vi "data_analysis main.vi"() -> ()   [LabVIEW 2017]
uses:
  <vilib>/Analysis/baseanly.llb/Mean (DBL).vi
  <vilib>/Waveform/WDTFileIO.llb/Export Waveforms To Spreadsheet File (1D).vi
  <vilib>/Analysis/NI_AALBase.lvlib
panel:
  out "x/y":dbl
  out "Zmag trajectory":waveform(dbl) caption="元素"
  out "Ext.":dbl
  out "Z pos":waveform(dbl)(graph)
  out "Zmag pos":waveform(dbl)(graph)
  out "data name":string
  out "cursor pos":dbl
  out "cursor length":dbl
  out "zmag cursor pos":dbl
  out "zmag cursor length":dbl
  out "current bead":string
  in  "graphs":enum32{"raw data", "force calculation"}(tab)
  out "XY图":cluster{dbl[], dbl[]}(graph)
  in  "ref NO.":i32 min=0
  in  "remove drift":bool
  in  "sample rate":dbl=200.0
  in  "zero point offset":bool
  out "x_0":dbl caption="X0" format="%0.2f"
  out "y_0":dbl caption="Y0" format="%0.2f"
  out "z_0":dbl caption="Z0" format="%0.2f"
  in  "file save path":path
  in  "数据另存为":bool
  in  "data type":enum16{"tdms", "gr", "excel"}(ring)
  out "保存完成？":bool
  in  "停止":bool
  in  "file path":path
  in  "load data":bool
  in  "data info":i32(listbox)
  in  "bead NO.":i32 min=0
  in  "trajectory":i32 min=0
  out "Z mag":dbl
  in  "zmag or force":enum32{"zmag", "force"}(radio)
  out "array of strings":string[](array[string])
  out "string":string
  in  "doubleFace?":bool
  in  "B":dbl=-1.436
  in  "A":dbl=142.6
  in  "cali source":enum32{"X", "Y"}(radio)
  out "Power spectrum (um^2/Hz)":cluster{dbl[], "Spectrum out":dbl[]}[](graph)
  in  "Z_shift":dbl
  out "Force graph":cluster{dbl[], dbl[]}(graph)
  in  "accept":bool
  in  "force estimate":bool
  in  "Fit settings":T1={"#PSD Averages"=40, "Correct camera acquisition artifacts"=TRUE, "Autorange"=TRUE, "fstart (Hz)"=0.0, "Pendulum geometry"=FALSE, "Fit model"=FALSE} {"#PSD Averages" min=1}
  in  "fsampling (Hz)":dbl=2800.0
  in  "DNA length (um)":dbl=0.658
  out "Fit Results":T2
  out "fit data":dbl[][](array[numeric])
  # "load force-zmag"
  # "F="
  # "exp(                *Zmag)"
  # "*"
  # "Fit parameters"
  # "Calculated quantities"
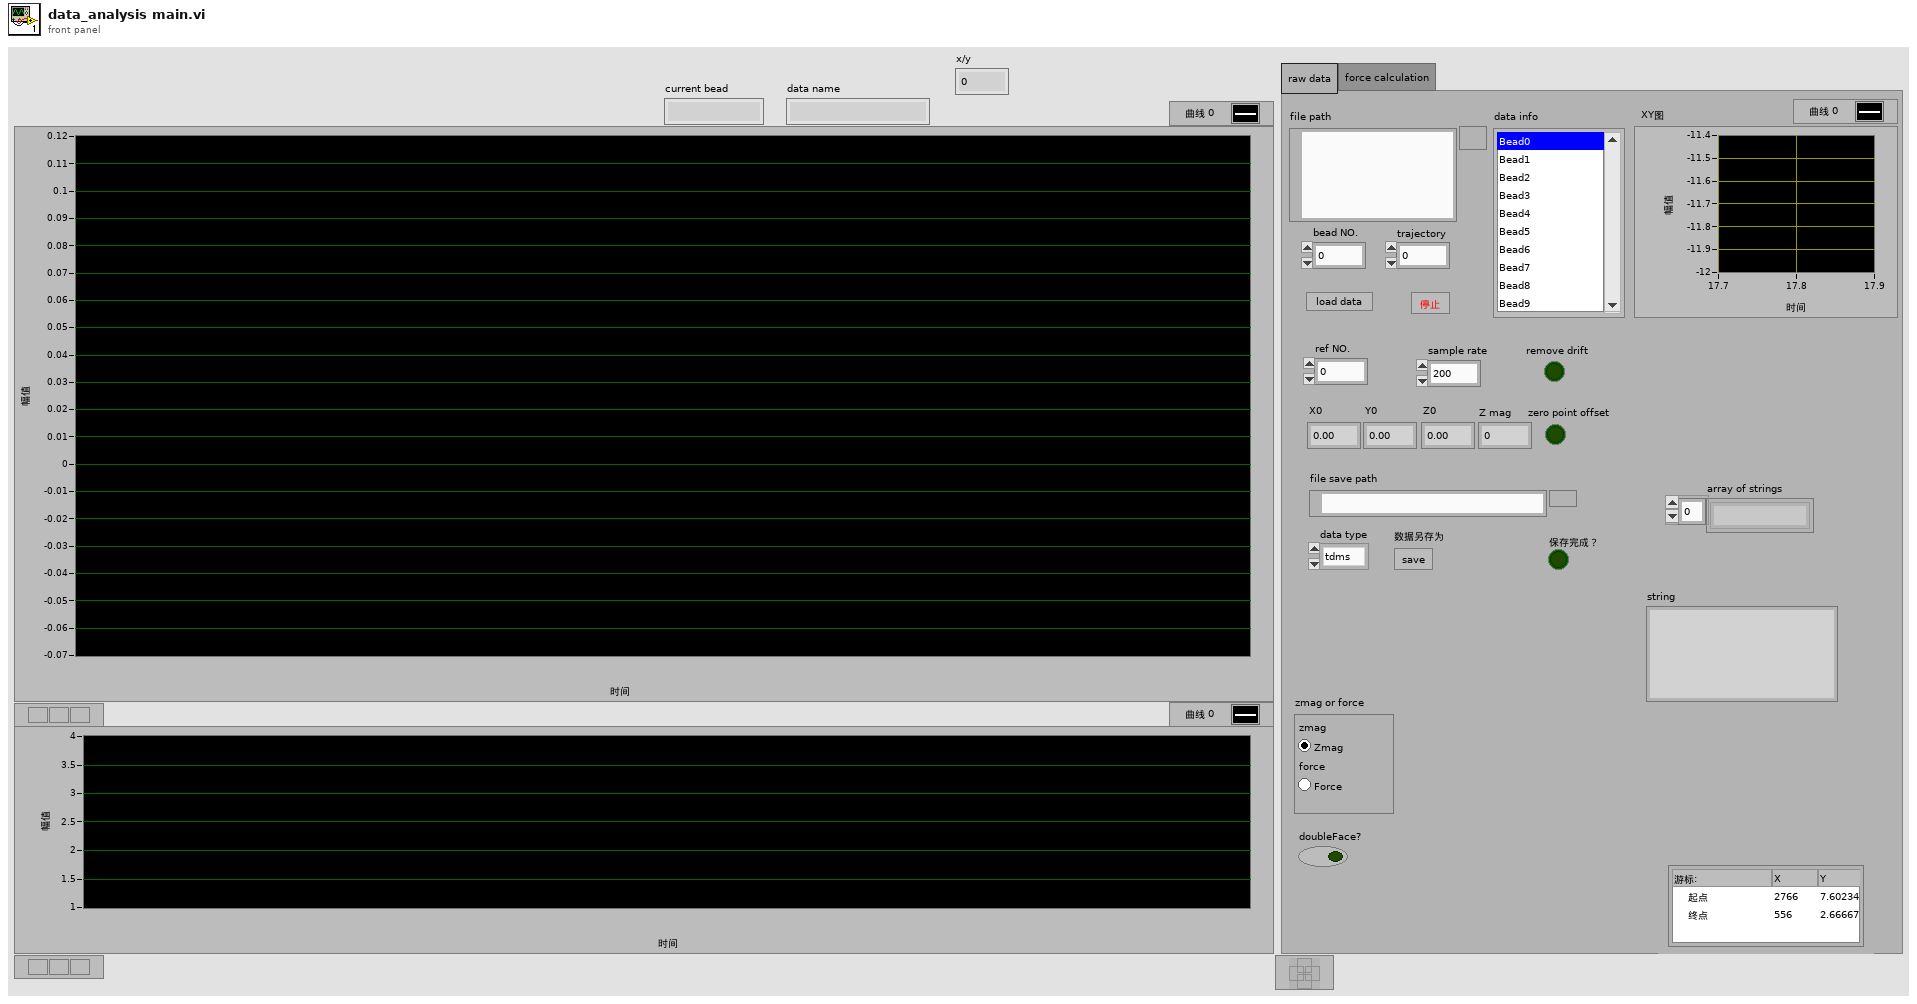
[diagram p1: front panel]
types:
  T1 = cluster{"#PSD Averages":u8, "Correct camera acquisition artifacts":bool, "Autorange":bool, "fstart (Hz)":dbl, "Pendulum geometry":bool, "Fit model":bool}
  T2 = cluster{"fcut (Hz)":dbl, "x2 (µm^2)":dbl, "Force (pN)":dbl, "Radius (µm)":dbl, "Apparent hydrodyn. radius (µm)":dbl, "fcut Error (Hz)":dbl, "x2 Error (µm^2)":dbl, "Force Error (pN)":dbl, "Radius Error (µm)":dbl, "Residue (unbiased)":dbl, "In range?":bool}
  T3 = enum16{"open", "open or create", "create or replace", "create", "open (read-only)"}
  T4 = enum16{"big-endian, network order", "native, host order", "little-endian"}
  T5 = enum16{"open", "replace", "create", "open or create", "replace or create", "replace or create with confirmation"}
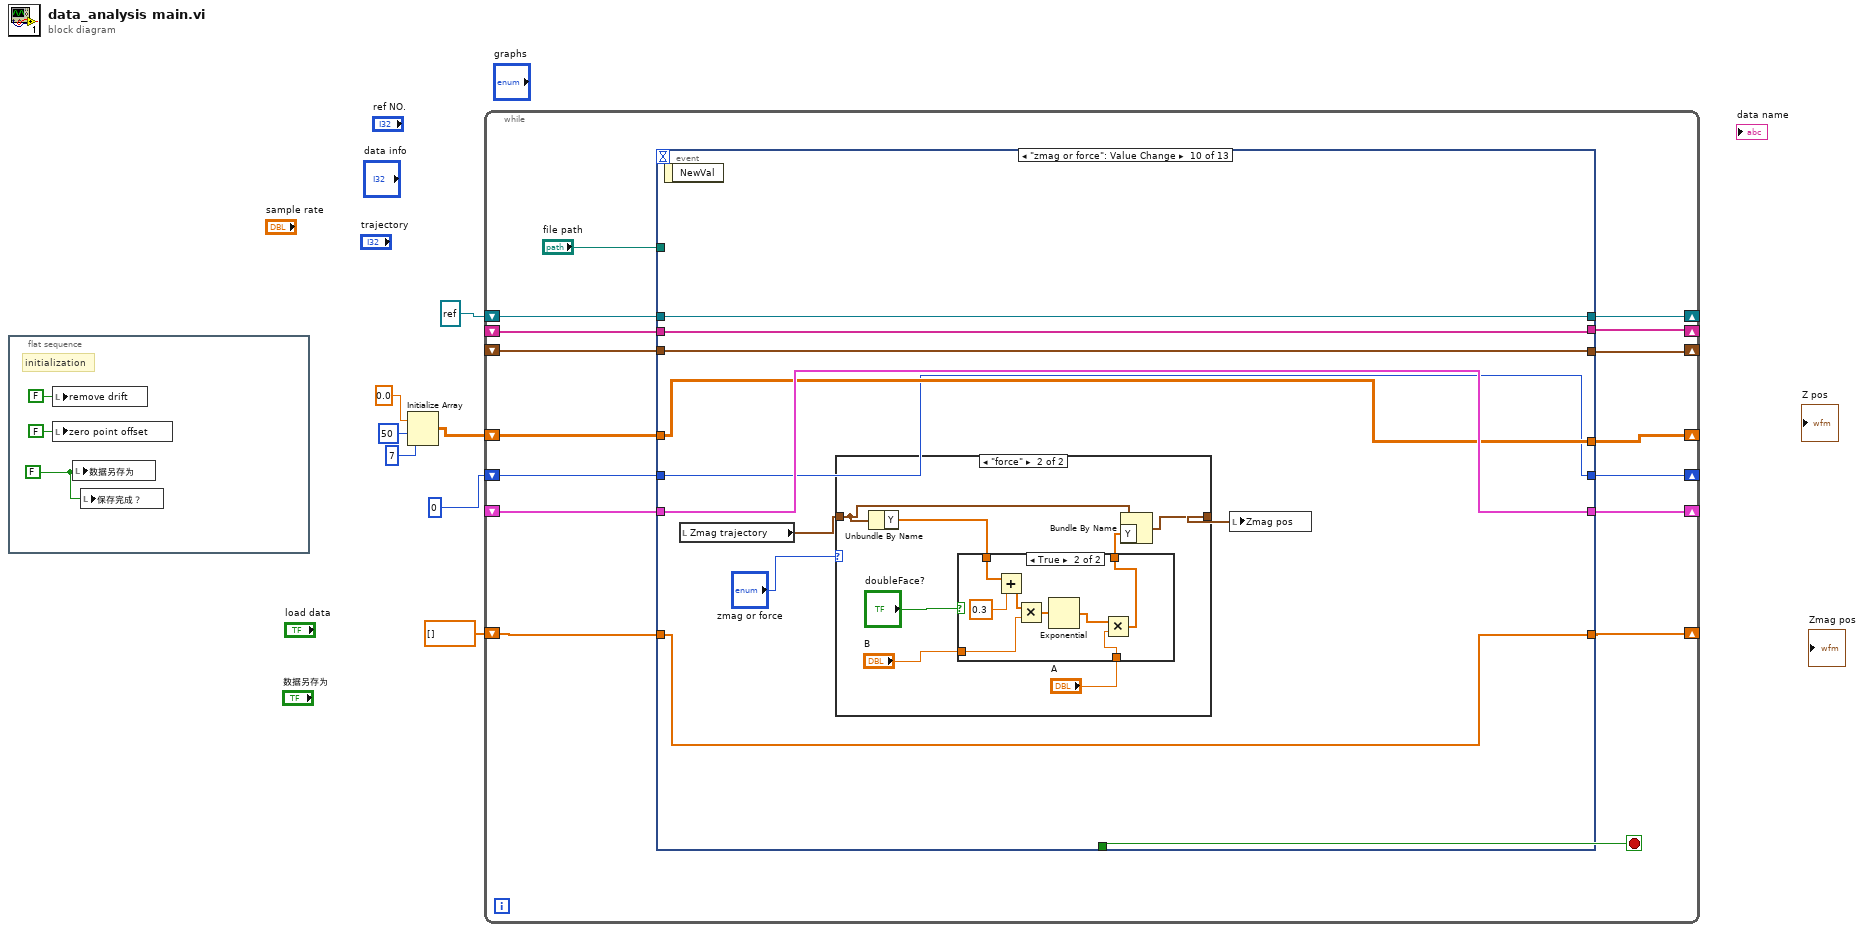
[diagram p0: block diagram]
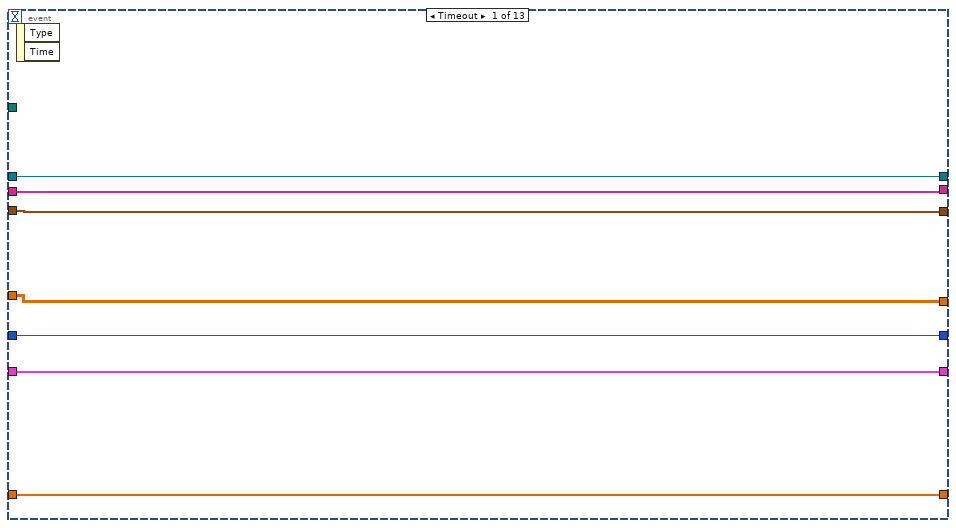
[diagram p2: hidden frame]
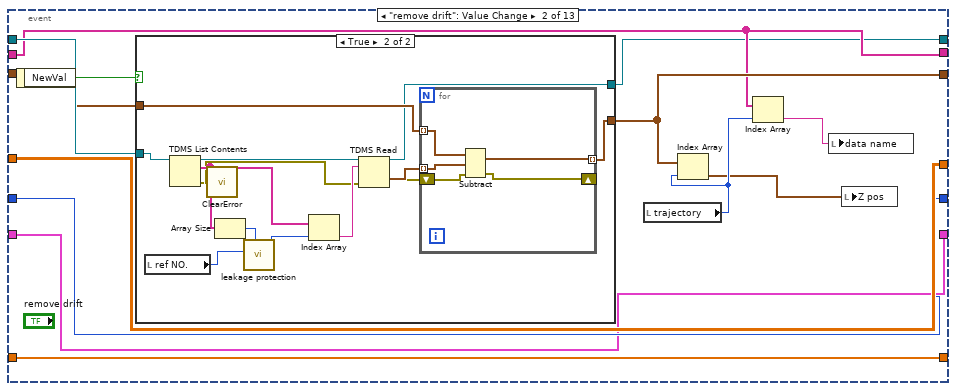
[diagram p3: hidden frame]
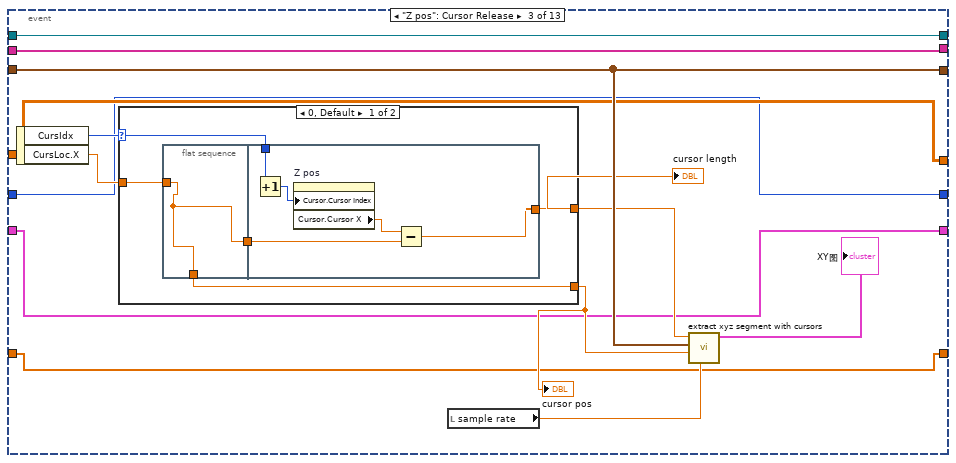
[diagram p5: hidden frame]
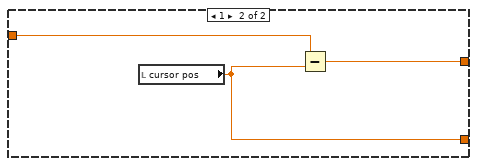
[diagram p6: hidden frame]
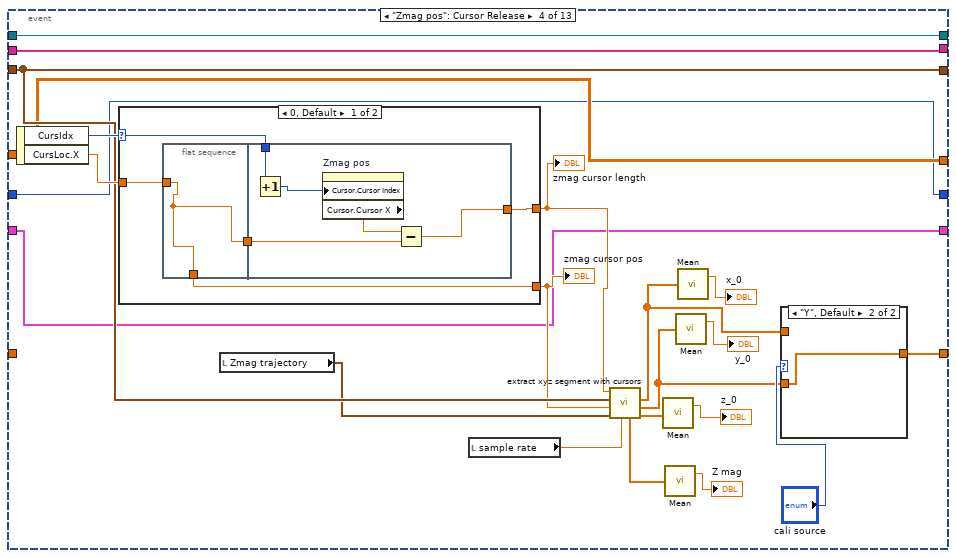
[diagram p7: hidden frame]
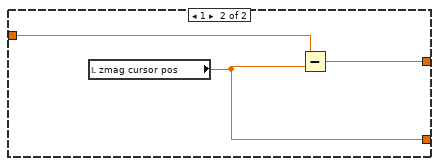
[diagram p9: hidden frame]
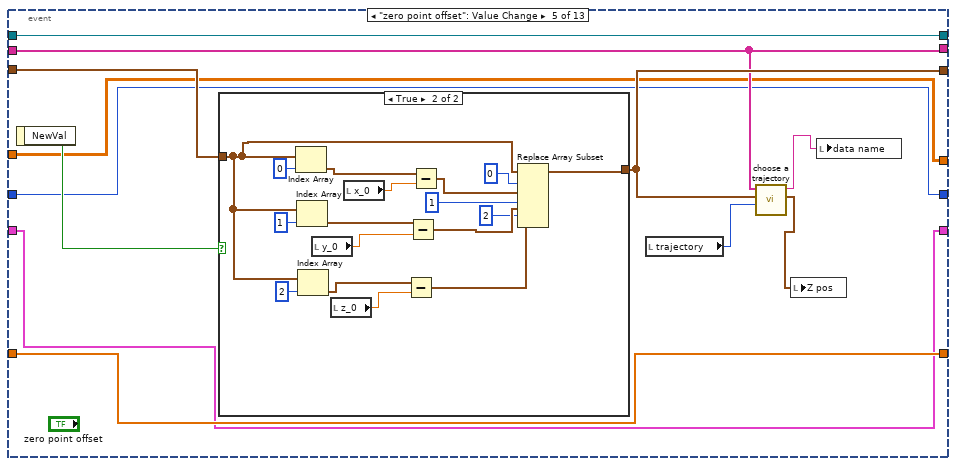
[diagram p10: hidden frame]
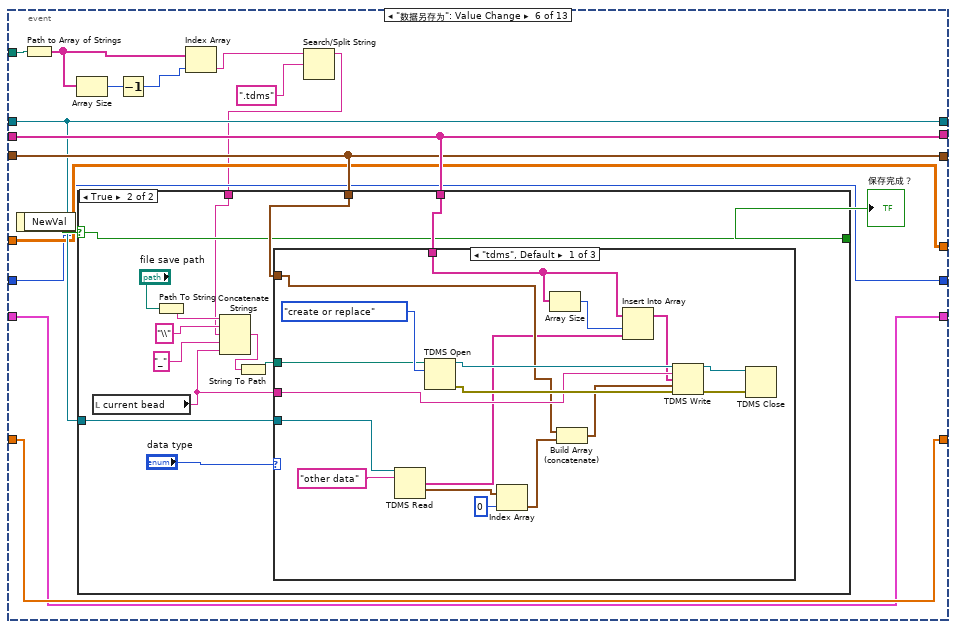
[diagram p12: hidden frame]
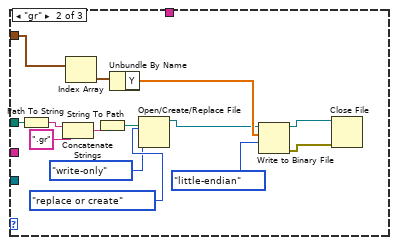
[diagram p14: hidden frame]
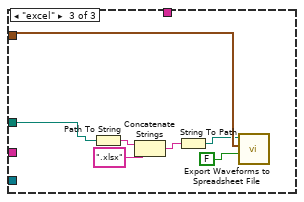
[diagram p15: hidden frame]
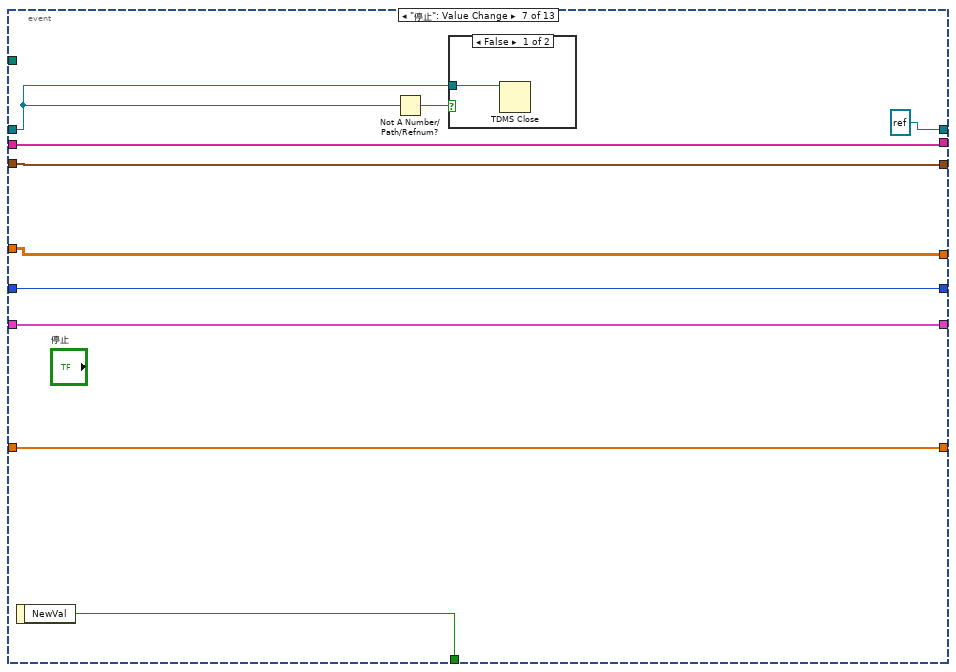
[diagram p16: hidden frame]
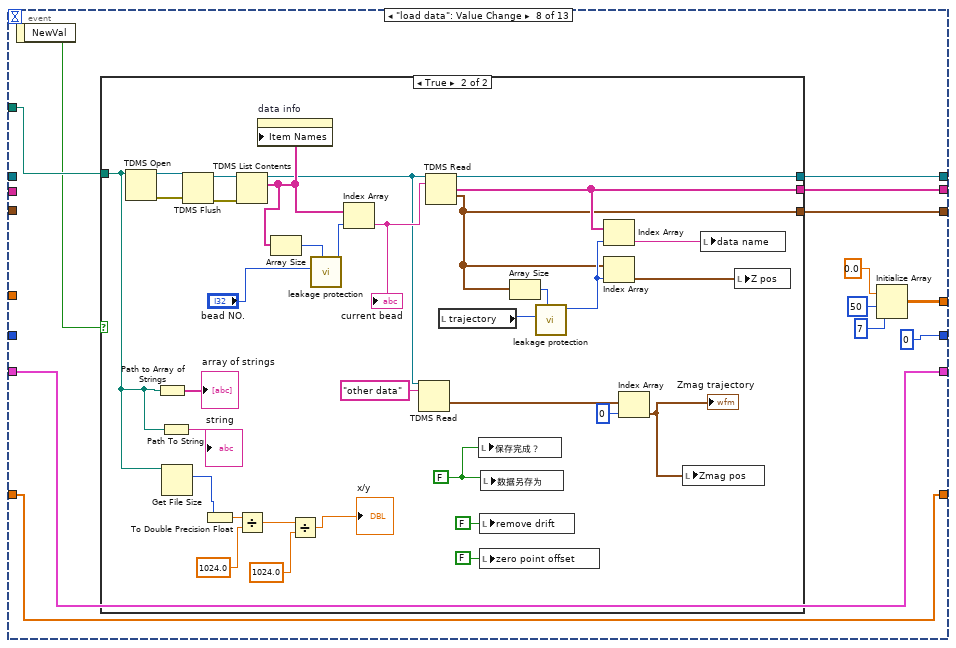
[diagram p18: hidden frame]
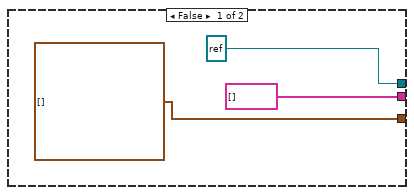
[diagram p19: hidden frame]
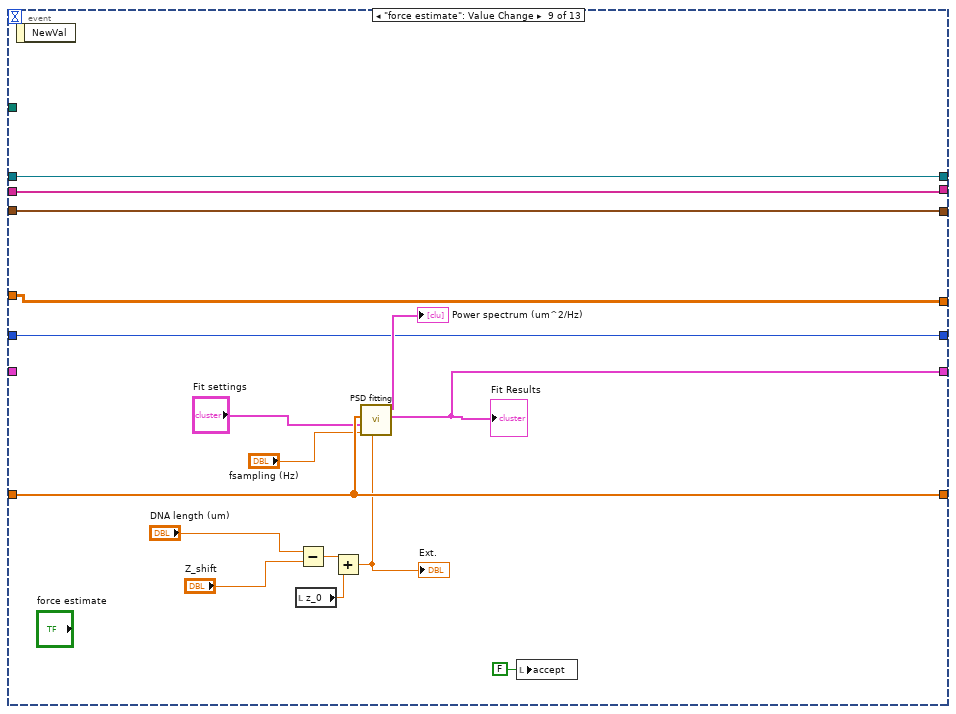
[diagram p20: hidden frame]
diagram:
  n1 = flat-sequence {
    frame #0 {
      w8 = FALSE ("数据另存为")
      # "initialization"
      n2 = local write "remove drift"(FALSE ("remove drift")) -> ()
      n3 = local write "zero point offset"(FALSE ("zero point offset")) -> ()
      n4 = local write "数据另存为"(w8) -> ()
      n5 = local write "保存完成？"(w8) -> ()
    }
  }
  n6 = Initialize Array(0.0 ("元素"), 50 ("维数大小"), 7 ("维数大小")) -> (w4:dbl[][])
  n7 = while {
    shift-right: [w24] -> _
    shift-left: refnum<k34> refnum ("tdms file out") -> [w19]
    shift-right: [w23] -> _
    shift-left: _ -> [w21]
    shift-right: [w22] -> _
    shift-left: _ -> [w20]
    shift-right: [w18] -> _
    shift-left: dbl[] [] ("Y") -> [w17]
    shift-right: [w16] -> _
    shift-left: _ -> [w15]
    shift-right: [w12] -> _
    shift-left: w4 -> [w14]
    shift-right: [w11] -> _
    shift-left: 0 -> [w13]
    stop <- w26 stop-if-true
    n8 = event shown="[9] \"zmag or force\": Value Change" {
      selector: _ -> [_ _ _ _ _ _ _ _ _ _ _ _ _]
      dyn-events: _ -> [_ _ _ _ _ _ _ _ _ _ _ _ _]
      timeout: _ -> [_ _ _ _ _ _ _ _ _ _ _ _ _]
      tunnel: [_ _ _ _ _ _ w241 _ _ _ _ _ _] -> w26
      tunnel: "file path" -> [_ _ _ _ _ w169 _ w254 _ _ _ _ _]
      tunnel: [w31 w40 w72 w105 w137 w174 refnum<k34> refnum ("tdms file out") w253 w307 w317 w358 refnum<k34> refnum ("tdms file out") w404] -> w24
      tunnel: [w33 w42 w80 w116 w140 w177 w240 w252 w306 w316 w357 w396 w405] -> w23
      tunnel: [w32 w43 w77 w113 w141 w176 w239 w251 w305 w315 w356 w395 w407] -> w22
      tunnel: w21 -> [w33 w42 w80 w116 w140 w177 w240 _ w306 w316 w357 w396 w405]
      tunnel: w20 -> [w32 w44 w77 w113 w143 w176 w239 _ w305 w315 w356 w395 w407]
      tunnel: w19 -> [w31 w45 w72 w105 w137 w174 w233 _ w307 w317 w358 w388 w404]
      tunnel: [w29 w37 w70 w96 w135 w172 w237 w249 w304 w314 w340 w392 w400] -> w18
      tunnel: w17 -> [w29 w37 w70 _ w135 w172 w237 w249 w304 w314 w340 w392 w400]
      tunnel: [w27 w35 w68 w102 w133 w170 w235 w248 w301 w313 w354 w390 w398] -> w16
      tunnel: w15 -> [w27 w35 w68 w102 w133 w170 w235 w248 _ w313 w354 w390 w398]
      tunnel: w14 -> [w30 w38 w71 w104 w136 w173 w238 _ w293 w312 w353 w393 w401]
      tunnel: w13 -> [w28 w36 w69 w103 w134 w171 w236 _ w292 w311 w352 w391 w399]
      tunnel: [w30 w38 w71 w104 w136 w173 w238 w244 w293 w312 w346 w393 w401] -> w12
      tunnel: [w28 w36 w69 w103 w134 w171 w236 0 w292 w311 w343 w391 w399] -> w11
      event Timeout {
        n9 = event-data() -> ()  [unwired: 1 in, 2 out]
      }
      event "remove drift": Value Change {
        n10 = event-data() -> ("NewVal"=w46:bool)  [unwired: 1 in]
        n11 = case shown="True" w46 {
          tunnel: w45 -> [w47 w57]
          tunnel: w44 -> [w48 w54]
          tunnel: [w48 w51] -> w43
          tunnel: [w47 w50] -> w40
          frame False {
          }
          frame True {
            n12 = local read "ref NO."() -> (w56:i32)
            n13 = TDMS List Contents(7:w57) -> (0:w49:errorcluster, 2:w60:string[], 3:w62:refnum<k34>)  [unwired: 2 in, 1 out]
            n14 = call <vilib>:"ClearError.vi"("error in (no error)"=w49) -> ("error out"=w55:errorcluster)
            n15 = Array Size(array=w60) -> (size(s)=w59:i32)
            n16 = call "leakage protection.vi"("matrix size"=w59, "index in"=w56) -> ("index out"=w58:i32)  [unwired: 9 in]
            n17 = Index Array(array=w60, index=w58) -> (element=w61:string)
            n18 = TDMS Read(0:w62, 5:w61, 11:w55) -> (4:w50:refnum<k34>, 10:w53:waveform(dbl)[], 15:w52:errorcluster)  [unwired: 5 in, 3 out]
            n19 = for {
              tunnel: w54 -> [w67] mode=indexing
              tunnel: w53 -> [w66] mode=indexing
              shift-right: [w64] -> _
              shift-left: w52 -> [w65]
              tunnel: [w63] -> w51 mode=indexing
              n20 = Subtract(1:w66, 2:w67, 4:w65) -> (0:w63:waveform(dbl), 3:w64:errorcluster)
            }
          }
        }
        n21 = local read "trajectory"() -> (w41:i32)
        n22 = Index Array(array=w43, index=w41) -> (element=w34:waveform(dbl))
        n23 = Index Array(array=w42, index=w41) -> (element=w39:string)
        n24 = local write "data name"(w39) -> ()
        n25 = local write "Z pos"(w34) -> ()
      }
      event "Z pos": Cursor Release {
        n26 = event-data() -> ("CursIdx"=w79:i32, "CursLoc.X"=w78:dbl)  [unwired: 1 in]
        n27 = case shown="0, Default" w79 {
          selector: w79 -> [w84 _]
          tunnel: w78 -> [w85 w94]
          tunnel: [w82 w93] -> w75
          tunnel: [w81 w92] -> w76
          frame 0, Default {
            n28 = flat-sequence {
              tunnel: w85 -> [w86]
              tunnel: [w86] -> w83
              tunnel: [w86] -> w81
              tunnel: w84 -> [w90]
              tunnel: w83 -> [w88]
              tunnel: [w87] -> w82
              frame #0 {
              }
              frame #1 {
                n29 = Increment(x=w90) -> (x+1=w91:i32)
                n30 = property on="Z pos" class="WFGraph (strict)"("Cursor.Cursor Index"=w91) -> ("Cursor.Cursor X"=w89:dbl)  [unwired: 2 in, 2 out]
                n31 = Subtract(x=w89, y=w88) -> (x-y=w87:dbl)
              }
            }
          }
          frame 1 {
            n32 = local read "cursor pos"() -> (w92:dbl)
            n33 = Subtract(x=w94, y=w92) -> (x-y=w93:dbl)
          }
        }
        "cursor length" <- w75
        "cursor pos" <- w76
        n34 = local read "sample rate"() -> (w74:dbl)
        n35 = call "extract xyz segment with cursors.vi"("sample rate"=w74, "cursor pos"=w76, "data"=w77, "cursor length"=w75) -> ("xy cluster"=→"XY图":cluster{dbl[], dbl[]})  [unwired: 3 in, 4 out]
      }
      event "Zmag pos": Cursor Release {
        n36 = event-data() -> ("CursIdx"=w115:i32, "CursLoc.X"=w114:dbl)  [unwired: 1 in]
        n37 = case shown="0, Default" w115 {
          selector: w115 -> [w122 _]
          tunnel: w114 -> [w123 w132]
          tunnel: [w120 w131] -> w111
          tunnel: [w119 w130] -> w112
          frame 0, Default {
            n38 = flat-sequence {
              tunnel: w123 -> [w124]
              tunnel: [w124] -> w121
              tunnel: [w124] -> w119
              tunnel: w122 -> [w129]
              tunnel: w121 -> [w128]
              tunnel: [w127] -> w120
              frame #0 {
              }
              frame #1 {
                n39 = Increment(x=w129) -> (x+1=w125:i32)
                n40 = property on="Zmag pos" class="WFGraph (strict)"("Cursor.Cursor Index"=w125) -> ("Cursor.Cursor X"=w126:dbl)  [unwired: 2 in, 2 out]
                n41 = Subtract(x=w126, y=w128) -> (x-y=w127:dbl)
              }
            }
          }
          frame 1 {
            n42 = local read "zmag cursor pos"() -> (w130:dbl)
            n43 = Subtract(x=w132, y=w130) -> (x-y=w131:dbl)
          }
        }
        "zmag cursor length" <- w111
        "zmag cursor pos" <- w112
        n44 = local read "Zmag trajectory"() -> (w101:waveform(dbl))
        n45 = local read "sample rate"() -> (w110:dbl)
        n46 = call "extract xyz segment with cursors.vi"("sample rate"=w110, "Zmag trajectory"=w101, "cursor pos"=w112, "data"=w113, "cursor length"=w111) -> ("Z"=w109:dbl[], "Y"=w97:dbl[], "X"=w95:dbl[], "Z mag"=w100:dbl[])  [unwired: 2 in, 1 out]
        n47 = call-poly <vilib>:"Mean.vi"("X"=w109) -> ("mean"=→"z_0":dbl)  [unwired: 1 out]
        n48 = call-poly <vilib>:"Mean.vi"("X"=w100) -> ("mean"=→"Z mag":dbl)  [unwired: 1 out]
        n49 = call-poly <vilib>:"Mean.vi"("X"=w97) -> ("mean"=→"y_0":dbl)  [unwired: 1 out]
        n50 = call-poly <vilib>:"Mean.vi"("X"=w95) -> ("mean"=→"x_0":dbl)  [unwired: 1 out]
        n51 = case shown="\"Y\", Default" "cali source" {
          tunnel: w97 -> [_ w118]
          tunnel: [w117 w118] -> w96
          tunnel: w95 -> [w117 _]
          frame "X" {
          }
          frame "Y", Default {
          }
        }
      }
      event "zero point offset": Value Change {
        n52 = event-data() -> ("NewVal"=w144:bool)  [unwired: 1 in]
        n53 = case shown="True" w144 {
          tunnel: w143 -> [w145 w151]
          tunnel: [w145 w146] -> w141
          frame False {
          }
          frame True {
            n54 = Index Array(array=w151, index=0 ("索引")) -> (element=w159:waveform(dbl))
            n55 = Index Array(array=w151, index=1 ("索引")) -> (element=w157:waveform(dbl))
            n56 = Index Array(array=w151, index=2 ("索引")) -> (element=w155:waveform(dbl))
            n57 = local read "y_0"() -> (w156:dbl)
            n58 = local read "z_0"() -> (w154:dbl)
            n59 = local read "x_0"() -> (w158:dbl)
            n60 = Subtract(x=w155, y=w154) -> (x-y=w147:waveform(dbl))
            n61 = Subtract(x=w157, y=w156) -> (x-y=w149:waveform(dbl))
            n62 = Subtract(x=w159, y=w158) -> (x-y=w152:waveform(dbl))
            n63 = Replace Array Subset(array=w151, new element #1=w152, index #1=0 ("索引"), new element #2=w149, index #2=1 ("索引"), new element #3=w147, index #3=2 ("索引")) -> (w146:waveform(dbl)[])
          }
        }
        n64 = local read "trajectory"() -> (w142:i32)
        n65 = call "choose a trajectory.vi"("trajectory"=w142, "data"=w141, "bead info"=w140) -> ("trajectory"=w139:waveform(dbl), "data name"=w138:string)  [unwired: 7 in]
        n66 = local write "Z pos"(w139) -> ()
        n67 = local write "data name"(w138) -> ()
      }
      event "数据另存为": Value Change {
        n68 = event-data() -> ("NewVal"=w178:bool)  [unwired: 1 in]
        n69 = Path to Array of Strings(0:w169) -> (2:w168:string[])  [unwired: 1 out]
        n70 = Array Size(array=w168) -> (size(s)=w167:i32)
        n71 = Decrement(x=w167) -> (x-1=w166:i32)
        n72 = Index Array(array=w168, index=w166) -> (element=w165:string)
        n73 = Search/Split String(string=w165, search string/char (-)=".tdms" ("搜索字符串/字符(-)")) -> (substring before match=w163:string)  [unwired: 1 in, 2 out]
        n74 = case shown="True" w178 {
          selector: w178 -> [w179 w184]
          tunnel: w177 -> [_ w192]
          tunnel: w176 -> [_ w191]
          tunnel: [w179 w184] -> w175
          tunnel: w174 -> [_ w183]
          tunnel: w163 -> [_ w182]
          frame False {
          }
          frame True {
            n75 = local read "current bead"() -> (w180:string)
            n76 = Path To String(path="file save path") -> (string=w189:string)
            n77 = Concatenate Strings(w189, "\\" ("字符串"), w182, "_" ("字符串"), w180) -> (w187:string)
            n78 = String To Path(string=w187) -> (path=w186:path)
            n79 = case shown="\"tdms\", Default" "data type" {
              tunnel: w192 -> [w196 _ _]
              tunnel: w191 -> [w199 w218 w231]
              tunnel: w186 -> [w207 w220 w229]
              tunnel: w180 -> [w204 _ _]
              tunnel: w183 -> [w200 _ _]
              frame "tdms", Default {
                n80 = TDMS Read(0:w200, 5:"other data" ("组名称输入")) -> (8:w195:string[], 10:w202:waveform(dbl)[])  [unwired: 6 in, 4 out]
                n81 = TDMS Open(10:T3."create or replace" ("操作(0:open)"), 11:w207) -> (0:w208:errorcluster, 3:w209:refnum<k34>)  [unwired: 5 in]
                n82 = Index Array(array=w202, index=0 ("索引")) -> (element=w198:waveform(dbl))
                n83 = Array Size(array=w196) -> (size(s)=w193:i32)
                n84 = Build Array (concatenate)(w199, w198) -> (w197:waveform(dbl)[])
                n85 = Insert Into Array(array=w196, index=w193, new element=w195) -> (w194:string[])
                n86 = TDMS Write(0:w209, 5:w204, 7:w194, 9:w197, 11:w208) -> (4:w206:refnum<k34>, 15:w205:errorcluster)  [unwired: 1 in, 2 out]
                n87 = TDMS Close(8:w205, 11:w206) -> ()  [unwired: 2 out]
              }
              frame "gr" {
                n88 = Path To String(path=w220) -> (string=w223:string)
                n89 = Concatenate Strings(w223, ".gr" ("字符串")) -> (w221:string)
                n90 = Index Array(array=w218) -> (element=w217:waveform(dbl))  [unwired: 1 in]
                n91 = String To Path(string=w221) -> (path=w219:path)
                n92 = Unbundle By Name(w217) -> ("Y"=w215:dbl[])
                n93 = Open/Create/Replace File(file path (use dialog)=w219, operation (0:open)=T5."replace or create" ("操作(0:open)"), access (0:read/write)=enum16{"read/write", "read-only", "write-only"}."write-only" ("权限(0:read/write)")) -> (refnum out=w214:refnum<file>)  [unwired: 3 in, 2 out]
                n94 = Write to Binary File(file (use dialog)=w214, data=w215, 9:T4."little-endian" ("字节顺序(0:big-endian, network order)")) -> (refnum out=w213:refnum<file>, error out=w212:errorcluster)  [unwired: 3 in, 1 out]
                n95 = Close File(refnum=w213, error in=w212) -> ()  [unwired: 2 out]
              }
              frame "excel" {
                n96 = Path To String(path=w229) -> (string=w228:string)
                n97 = Concatenate Strings(w228, ".xlsx" ("字符串")) -> (w226:string)
                n98 = String To Path(string=w226) -> (path=w225:path)
                n99 = call-poly <vilib>:"Export Waveforms to Spreadsheet File.vi"("multiple time columns? (single:F)"=FALSE ("append to file? (new file:F)"), "waveforms"=w231, "file path (dialog if empty)"=w225) -> ()  [unwired: 7 in, 2 out]
              }
            }
          }
        }
        "保存完成？" <- w175
      }
      event "停止": Value Change {
        n100 = event-data() -> ("NewVal"=w241:bool)  [unwired: 1 in]
        n101 = Not A Number/Path/Refnum?(number/path/refnum=w233) -> (NaN/Path/Refnum?=w234:bool)
        n102 = case shown="False" w234 {
          tunnel: w233 -> [w242 _]
          frame False {
            n103 = TDMS Close(11:w242) -> ()  [unwired: 1 in, 2 out]
          }
          frame True {
          }
        }
      }
      event "load data": Value Change {
        n104 = event-data() -> ("NewVal"=w250:bool)  [unwired: 1 in]
        n105 = case shown="True" w250 {
          tunnel: w254 -> [_ w259]
          tunnel: [refnum<k34> refnum ("tdms file out") w290] -> w253
          tunnel: [string[] [] ("channel name(s) out") w289] -> w252
          tunnel: [waveform(dbl)[] [] ("data") w282] -> w251
          frame False {
          }
          frame True {
            w267 = FALSE ("数据另存为")
            n106 = TDMS Open(11:w259) -> (0:w278:errorcluster, 3:w279:refnum<k34>)  [unwired: 6 in]
            n107 = Path to Array of Strings(0:w259) -> (2:→"array of strings":string[])  [unwired: 1 out]
            n108 = Path To String(path=w259) -> (string=→"string":string)
            n109 = Get File Size(file=w259) -> (size (in bytes)=w266:i64)  [unwired: 1 in, 2 out]
            n110 = TDMS Flush(4:w278, 7:w279) -> (0:w277:errorcluster, 3:w276:refnum<k34>)
            n111 = To Double Precision Float(number=w266) -> (double precision float=w265:dbl)
            n112 = TDMS List Contents(4:w277, 7:w276) -> (2:w286:string[], 3:w275:refnum<k34>)  [unwired: 1 in, 2 out]
            n113 = Divide(x=w265, y=1024.0) -> (x/y=w262:dbl)
            n114 = property on="data info" class="LstBox (strict)"("Item Names"=w286) -> ()  [unwired: 2 in, 2 out]
            n115 = Array Size(array=w286) -> (size(s)=w285:i32)
            n116 = Divide(x=w262, y=1024.0) -> (x/y=→"x/y":dbl)
            n117 = call "leakage protection.vi"("matrix size"=w285, "index in"="bead NO.") -> ("index out"=w284:i32)  [unwired: 9 in]
            n118 = Index Array(array=w286, index=w284) -> (element=w291:string)
            "current bead" <- w291
            n119 = TDMS Read(0:w275, 5:"other data" ("组名称输入")) -> (10:w273:waveform(dbl)[])  [unwired: 6 in, 5 out]
            n120 = TDMS Read(0:w275, 5:w291) -> (4:w290:refnum<k34>, 8:w289:string[], 10:w282:waveform(dbl)[])  [unwired: 6 in, 3 out]
            n121 = local read "trajectory"() -> (w283:i32)
            n122 = local write "保存完成？"(w267) -> ()
            n123 = local write "remove drift"(FALSE ("remove drift")) -> ()
            n124 = local write "zero point offset"(FALSE ("zero point offset")) -> ()
            n125 = local write "数据另存为"(w267) -> ()
            n126 = Array Size(array=w282) -> (size(s)=w287:i32)
            n127 = call "leakage protection.vi"("matrix size"=w287, "index in"=w283) -> ("index out"=w288:i32)  [unwired: 9 in]
            n128 = Index Array(array=w289, index=w288) -> (element=w281:string)
            n129 = Index Array(array=w282, index=w288) -> (element=w280:waveform(dbl))
            n130 = Index Array(array=w273, index=0 ("索引")) -> (element=w268:waveform(dbl))
            "Zmag trajectory" <- w268
            n131 = local write "Zmag pos"(w268) -> ()
            n132 = local write "data name"(w281) -> ()
            n133 = local write "Z pos"(w280) -> ()
          }
        }
        n134 = Initialize Array(0.0 ("元素"), 50 ("维数大小"), 7 ("维数大小")) -> (w244:dbl[][])
      }
      event "force estimate": Value Change {
        n135 = event-data() -> ()  [unwired: 1 in, 1 out]
        n136 = local read "z_0"() -> (w296:dbl)
        n137 = Subtract(x="DNA length (um)", y="Z_shift") -> (x-y=w297:dbl)
        n138 = Add(x=w297, y=w296) -> (x+y=w295:dbl)
        "Ext." <- w295
        n139 = call "PSD fitting.vi"("DNA length (µm)"=w295, "fsampling (Hz)"="fsampling (Hz)", "Fit settings"="Fit settings", "X/Y data"=w304) -> ("Fit Results"=w301:T2, "Power spectrum (um^2/Hz)"=→"Power spectrum (um^2/Hz)":cluster{dbl[], "Spectrum out":dbl[]}[])  [unwired: 6 in]
        "Fit Results" <- w301
        n140 = local write "accept"(FALSE ("accept")) -> ()
      }
      event "zmag or force": Value Change {
        n141 = event-data() -> ()  [unwired: 1 in, 1 out]
        n142 = local read "Zmag trajectory"() -> (w309:waveform(dbl))
        n143 = case shown="\"force\"" "zmag or force" {
          tunnel: w309 -> [w318 w322]
          tunnel: [w318 w324] -> w308
          frame "zmag", Default {
          }
          frame "force" {
            n144 = Unbundle By Name(w322) -> ("Y"=w325:dbl[])
            n145 = case shown="True" "doubleFace?" {
              tunnel: w325 -> [w331 w334]
              tunnel: [w328 w332] -> w323
              tunnel: "B" -> [w327 w337]
              tunnel: "A" -> [w326 w336]
              frame False {
                n146 = Multiply(x=w331, y=w327) -> (x*y=w330:dbl[])
                n147 = Exponential(1:w330) -> (0:w329:dbl[])
                n148 = Multiply(x=w329, y=w326) -> (x*y=w328:dbl[])
              }
              frame True {
                n149 = Add(x=w334, y=0.3) -> (x+y=w335:dbl[])
                n150 = Multiply(x=w335, y=w337) -> (x*y=w339:dbl[])
                n151 = Exponential(1:w339) -> (0:w338:dbl[])
                n152 = Multiply(x=w338, y=w336) -> (x*y=w332:dbl[])
              }
            }
            n153 = Bundle By Name(cluster=w322, "Y"=w323) -> (w324:waveform(dbl))
          }
        }
        n154 = local write "Zmag pos"(w308) -> ()
      }
      event "accept": Value Change {
        n155 = event-data() -> ()  [unwired: 1 in, 1 out]
        n156 = case shown="True" "accept" {
          tunnel: w354 -> [_ w385]
          tunnel: w353 -> [w359 w371]
          tunnel: w352 -> [w360 w363]
          tunnel: [w359 w361] -> w346
          tunnel: [w360 w373] -> w343
          frame False {
          }
          frame True {
            n157 = Unbundle By Name(w385) -> ("Force (pN)"=w384:dbl, "Force Error (pN)"=w379:dbl, "Radius (µm)"=w378:dbl, "Radius Error (µm)"=w377:dbl, "fcut (Hz)"=w364:dbl)
            n158 = local read "Z mag"() -> (w367:dbl)
            n159 = local read "Ext."() -> (w369:dbl)
            n160 = Replace Array Subset(array=w371, new element=w369, index (row)=w363, index (col)=0 ("禁用的索引 (列)")) -> (w370:dbl[][])
            n161 = Replace Array Subset(array=w370, new element=w384, index (row)=w363, index (col)=1 ("禁用的索引 (列)")) -> (w376:dbl[][])
            n162 = Replace Array Subset(array=w376, new element=w379, index (row)=w363, index (col)=2 ("禁用的索引 (列)")) -> (w375:dbl[][])
            n163 = Replace Array Subset(array=w375, new element=w378, index (row)=w363, index (col)=3 ("禁用的索引 (列)")) -> (w374:dbl[][])
            n164 = Replace Array Subset(array=w374, new element=w377, index (row)=w363, index (col)=4 ("禁用的索引 (列)")) -> (w366:dbl[][])
            n165 = Replace Array Subset(array=w366, new element=w367, index (row)=w363, index (col)=5 ("禁用的索引 (列)")) -> (w362:dbl[][])
            n166 = Replace Array Subset(array=w362, new element=w364, index (row)=w363, index (col)=6 ("禁用的索引 (列)")) -> (w361:dbl[][])
            n167 = Increment(x=w363) -> (x+1=w373:i32)
          }
        }
        n168 = Array Subset(array=w346, index (row)=0 ("索引"), length (row)=w343, index (col)=0 ("索引"), length (col)=7 ("长度")) -> (w341:dbl[][])
        "fit data" <- w341
        n169 = Index Array(array=w341, index (col) #1=0 ("禁用的索引 (列)"), index (col) #2=1 ("索引 (列)")) -> (element #1=w350:dbl[], element #2=w348:dbl[])  [unwired: 2 in]
        n170 = Bundle(w350, w348) -> (→"Force graph":cluster{dbl[], dbl[]})  [unwired: 1 in]
      }
      event "file path": Value Change {
        n171 = event-data() -> ("NewVal"=w394:path)  [unwired: 1 in, 4 out]
        n172 = local write "file path"(w394) -> ()
        n173 = local write "bead NO."(0 ("bead NO.")) -> ()
        n174 = Not A Number/Path/Refnum?(number/path/refnum=w388) -> (NaN/Path/Refnum?=w387:bool)
        n175 = case shown="True" w387 {
          tunnel: w388 -> [w397 _]
          frame False {
            n176 = TDMS Close(11:w397) -> ()  [unwired: 1 in, 2 out]
          }
          frame True {
          }
        }
      }
      event "trajectory": Value Change {
        n177 = event-data() -> ("NewVal"=w406:i32)  [unwired: 1 in]
        n178 = call "choose a trajectory.vi"("trajectory"=w406, "data"=w407, "bead info"=w405) -> ("trajectory"=w402:waveform(dbl), "data name"=w403:string)  [unwired: 7 in]
        n179 = local write "data name"(w403) -> ()
        n180 = local write "Z pos"(w402) -> ()
      }
    }
  }
